vi "SMR_LabVIEW_V4.vi"() -> ()   [LabVIEW 2025]
uses:
  <vilib>/DAQmx/write.llb/DAQmx Write (Analog DBL 1Chan 1Samp).vi
  <vilib>/DAQmx/read.llb/DAQmx Read (Analog 1D DBL NChan 1Samp).vi
  <vilib>/DAQmx/create/channels.llb/DAQmx Create Channel (AI-Temperature-Thermocouple).vi
  <vilib>/DAQmx/create/channels.llb/DAQmx Create Channel (AI-Voltage-Basic).vi
  <vilib>/DAQmx/create/channels.llb/DAQmx Create Channel (AO-Voltage-Basic).vi
  <vilib>/DAQmx/miscellaneous.llb/DAQmx Fill In Error Info.vi
panel:
  in  "Shutdown Valve Command (%)":dbl min=0.0 max=100.0
  out "Valve Command Before Enable (%)":dbl
  out "Valve Output Voltage (V)":dbl
  out "Valve Command Final (%)":dbl
  in  "Valve Output Enable":bool
  in  "Manual Valve Command (%)":dbl min=0.0 max=100.0
  out "Heat Exchanger Pressure History":dbl(graph)
  out "Main Loop Pressure History":T1(graph)
  out "Heat Exchanger Temperature History":cluster{"Waveform":dbl, "Waveform":dbl}(graph)
  out "Main Loop Temeperature History":T2(graph)
  out "Overall Avg Pressure (psi)":dbl
  out "Heat Exchanger Pressure P6 (psi)":dbl
  out "Main Loop Avg Pressure (psi)":dbl
  out "Heat Exchanger Avg Temp (deg C)":dbl
  out "Main Loop Avg Temp (deg C)":dbl
  out "Raw NI9201 \nVoltage Display":T3
  out "Temperature Display":T4
  out "Pressure Display":T5
  in  "Flow Offset Correction (GPM)":dbl=-0.3
  out "Flow History":dbl(graph)
  out "Overall Pressure History":T6(graph)
  out "Overall Temperature History":T7(graph)
  out "Max Loop Pressure (psi)":dbl
  out "Overall Avg Temp (deg C)":dbl
  out "Max Loop Temp (deg C)":dbl
  out "Heat Exchanger Flow (GPM)":dbl
  in  "Loop Period (ms)":dbl=1000.0
  in  "Stop":bool
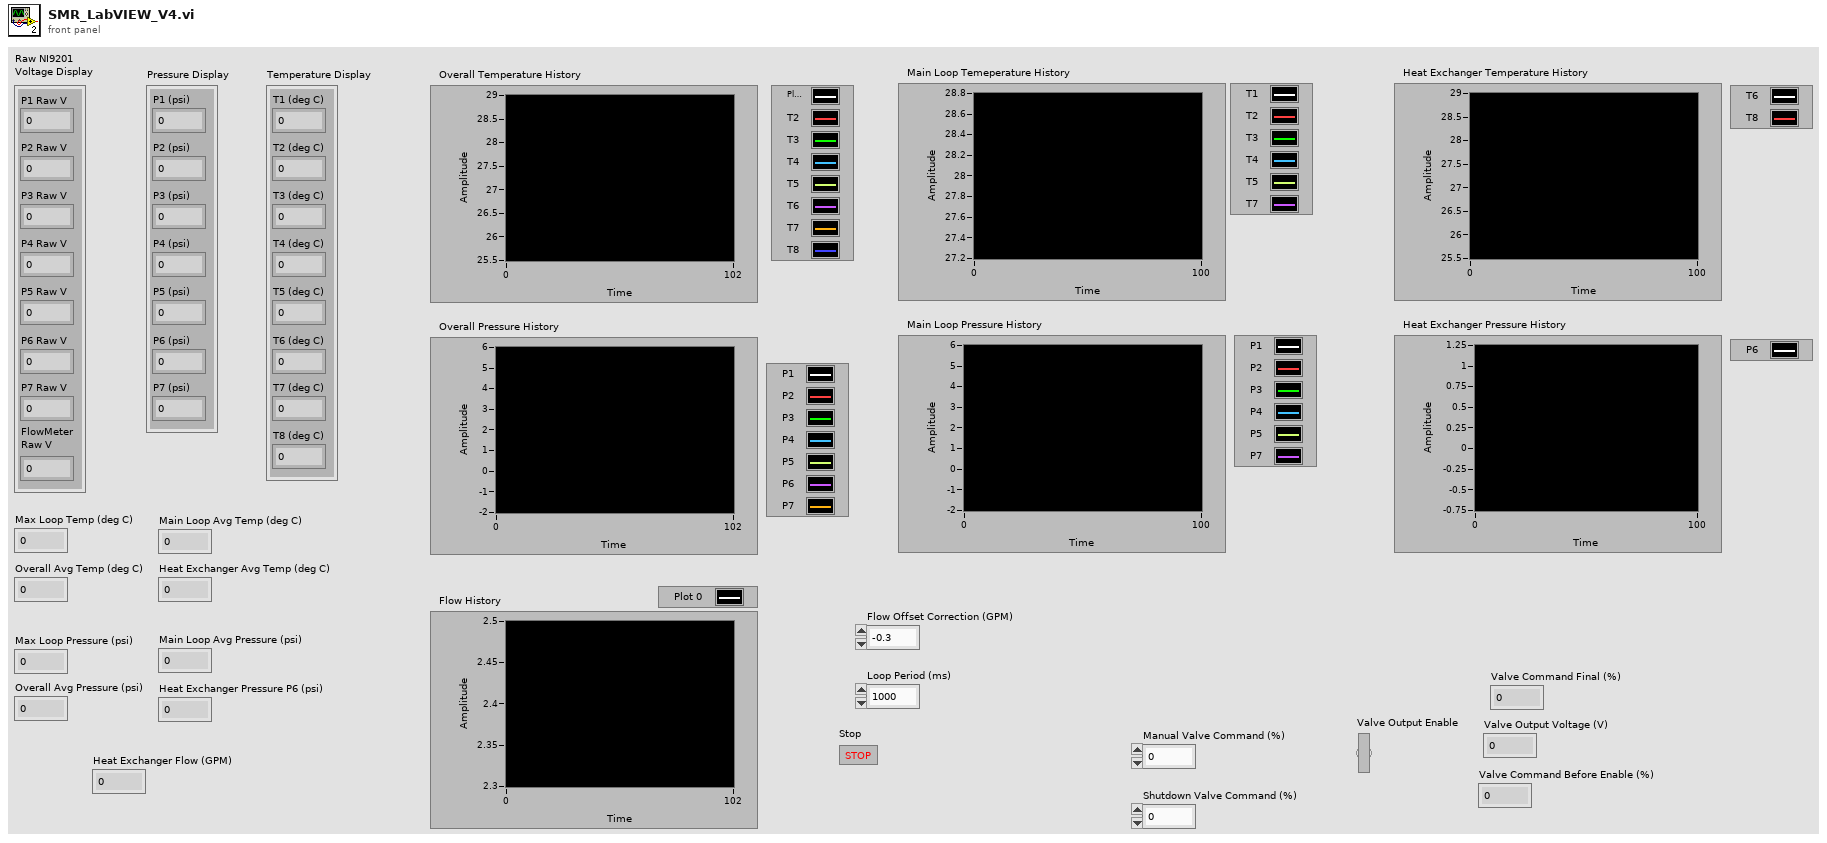
[diagram p1: front panel]
types:
  T1 = cluster{"P1":dbl, "P2":dbl, "P3":dbl, "P4":dbl, "P5":dbl, "P7":dbl}
  T2 = cluster{"Waveform":dbl, "Waveform":dbl, "Waveform":dbl, "Waveform":dbl, "Waveform":dbl, "Waveform":dbl}
  T3 = cluster{"P1 Raw V":dbl, "P2 Raw V":dbl, "P3 Raw V":dbl, "P4 Raw V":dbl, "P5 Raw V":dbl, "P6 Raw V":dbl, "P7 Raw V":dbl, "FlowMeter\nRaw V":dbl}
  T4 = cluster{"T1 (deg C)":dbl, "T2 (deg C)":dbl, "T3 (deg C)":dbl, "T4 (deg C)":dbl, "T5 (deg C)":dbl, "T6 (deg C)":dbl, "T7 (deg C)":dbl, "T8 (deg C)":dbl}
  T5 = cluster{"P1 (psi)":dbl, "P2 (psi)":dbl, "P3 (psi)":dbl, "P4 (psi)":dbl, "P5 (psi)":dbl, "P6 (psi)":dbl, "P7 (psi)":dbl}
  T6 = cluster{"P1":dbl, "P2":dbl, "P3":dbl, "P4":dbl, "P5":dbl, "P6":dbl, "P7":dbl}
  T7 = cluster{"Waveform":dbl, "Waveform":dbl, "Waveform":dbl, "Waveform":dbl, "Waveform":dbl, "Waveform":dbl, "Waveform":dbl, "Waveform":dbl}
  T8 = cluster{"P1":dbl, "P2":dbl, "P3":dbl, "P4":dbl, "P5":dbl, "P6":dbl, "P7":dbl, "Flow":dbl}
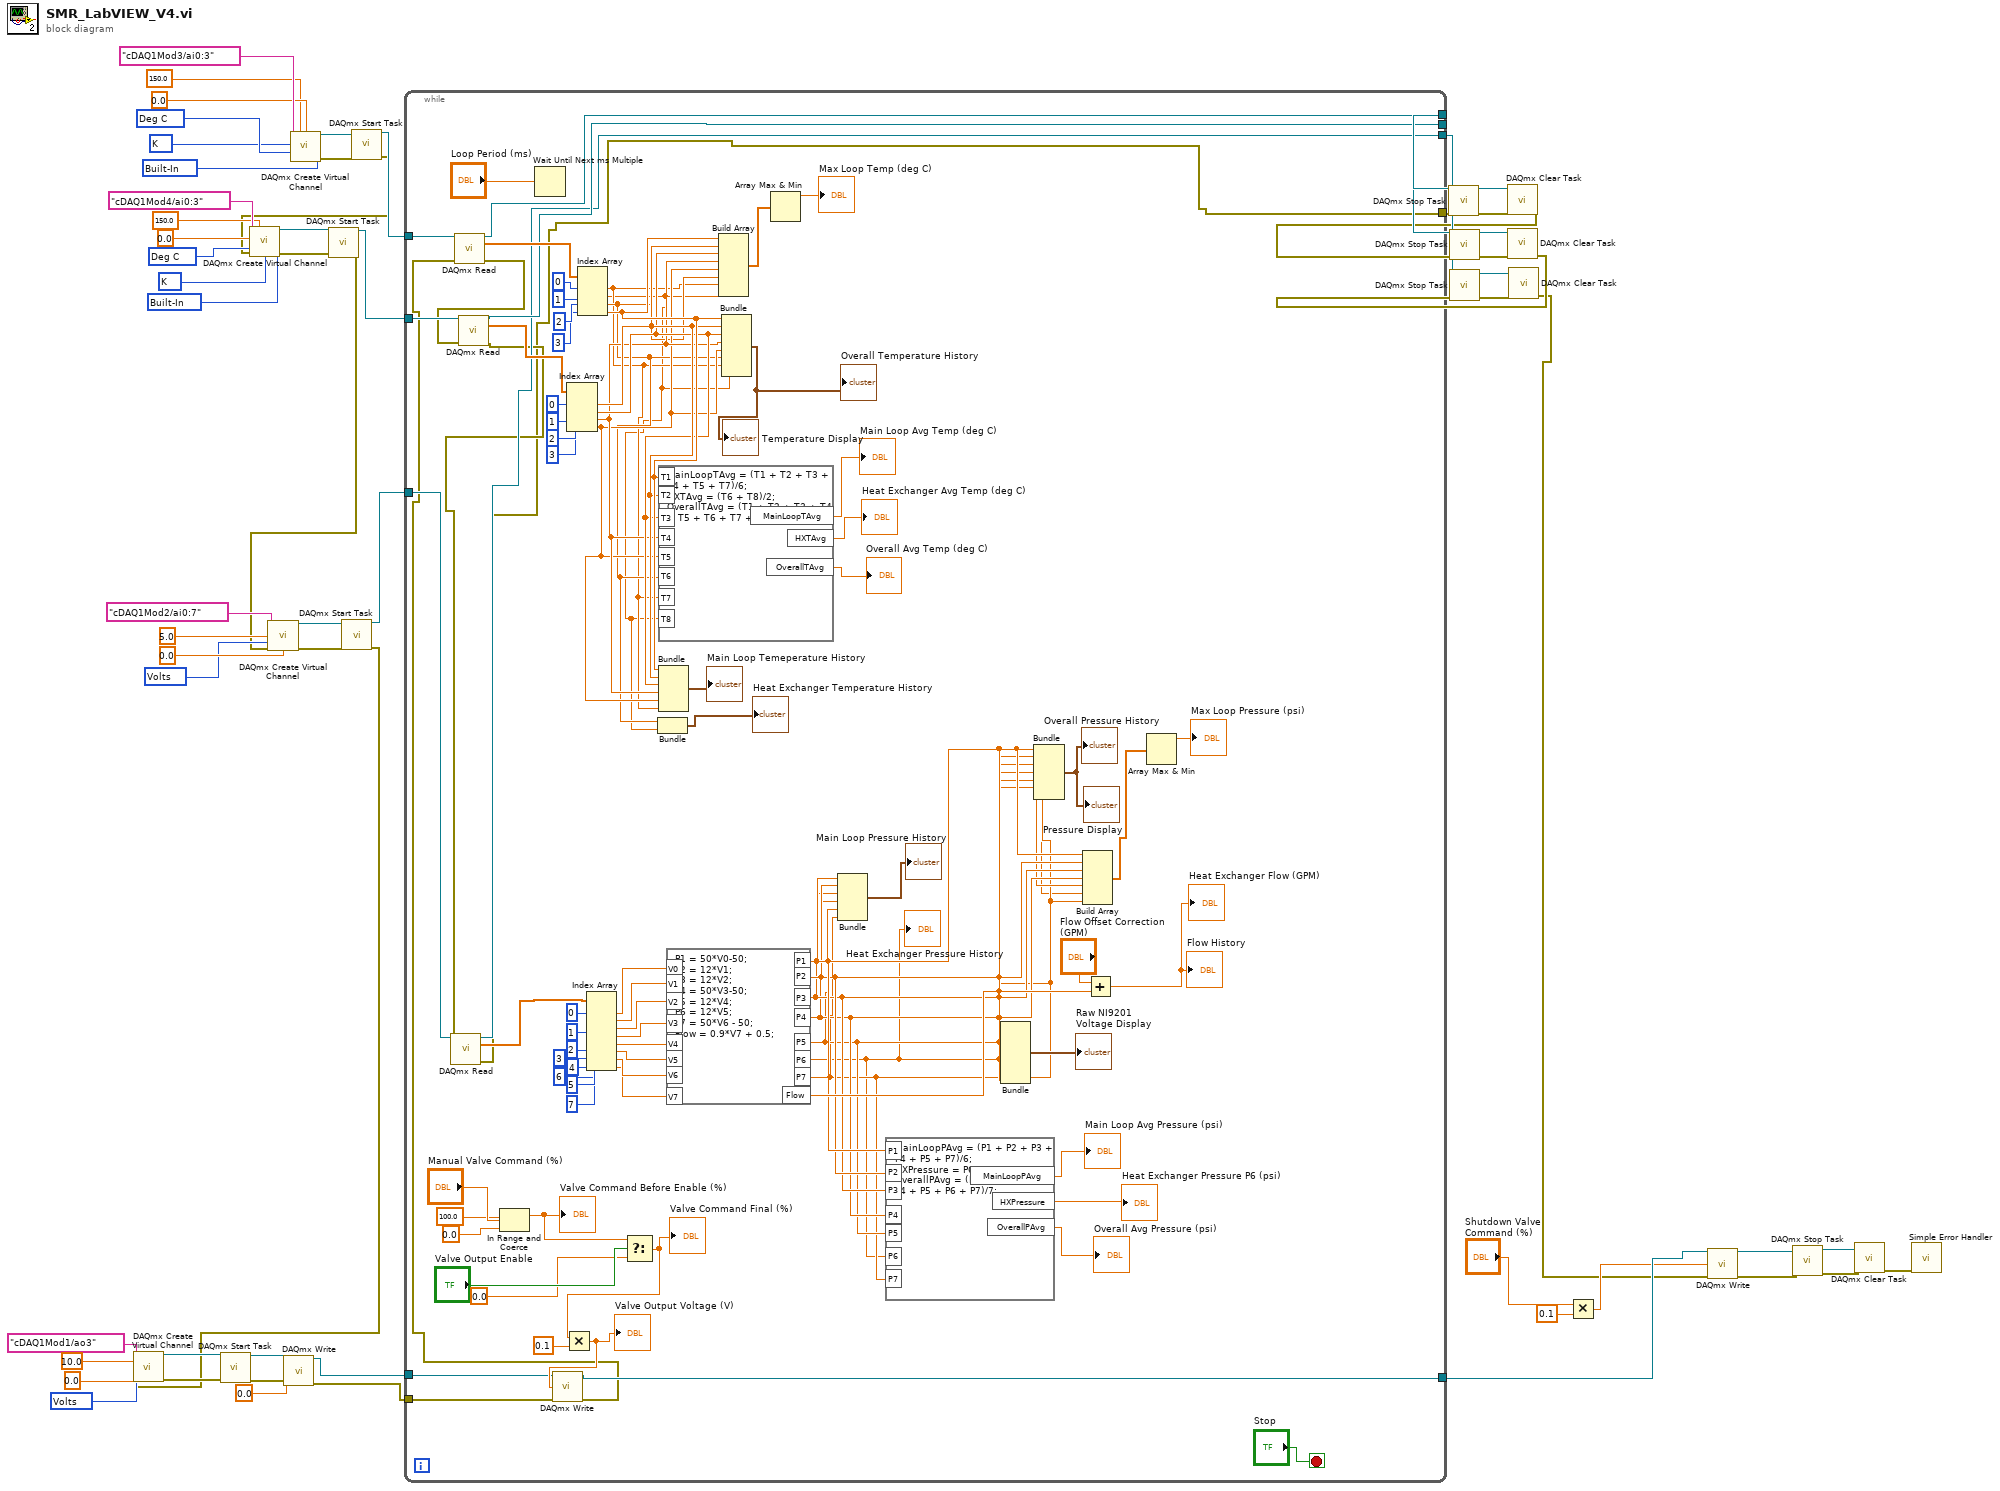
[diagram p0: block diagram]
diagram:
  w19 = 10348 items=["Volts"=10348, "From Custom Scale"=10065] ("units")
  w43 = 10348 items=["Volts"=10348, "From Custom Scale"=10065] ("units")
  w47 = 10200 items=["Built-In"=10200, "Constant Value"=10116, "Channel"=10113] ("cjc source")
  w48 = 10073 items=["J"=10072, "K"=10073, "N"=10077, "R"=10082, "S"=10085, "T"=10086, "B"=10047, "E"=10055] ("thermocouple type")
  w31 = 10143 items=["Deg C"=10143, "Deg F"=10144, "Kelvins"=10325, "Deg R"=10145, "From Custom Scale"=10065] ("units")
  w51 = 10200 items=["Built-In"=10200, "Constant Value"=10116, "Channel"=10113] ("cjc source")
  w52 = 10073 items=["J"=10072, "K"=10073, "N"=10077, "R"=10082, "S"=10085, "T"=10086, "B"=10047, "E"=10055] ("thermocouple type")
  w55 = 10143 items=["Deg C"=10143, "Deg F"=10144, "Kelvins"=10325, "Deg R"=10145, "From Custom Scale"=10065] ("units")
  n1 = call-poly <vilib>:"DAQmx Create Virtual Channel.vi"("maximum value"=150.0, "minimum value"=0.0, "physical channels"=tag "cDAQ1Mod3/ai0:3", "cjc source"=w51, "units"=w55, "thermocouple type"=w52) -> ("task out"=w60:refnum<k21>, "error out"=w59:errorcluster)  [unwired: 8 in]
  n2 = call <vilib>:"DAQmx Start Task.vi"("task/channels in"=w60, "error in"=w59) -> ("task out"=w40:refnum<k21>, "error out"=w30:errorcluster)  [unwired: 12 in]
  n3 = call-poly <vilib>:"DAQmx Create Virtual Channel.vi"("maximum value"=150.0, "minimum value"=0.0, "physical channels"=tag "cDAQ1Mod4/ai0:3", "cjc source"=w47, "units"=w31, "error in"=w30, "thermocouple type"=w48) -> ("task out"=w57:refnum<k21>, "error out"=w56:errorcluster)  [unwired: 7 in]
  n4 = call <vilib>:"DAQmx Start Task.vi"("task/channels in"=w57, "error in"=w56) -> ("task out"=w39:refnum<k21>, "error out"=w29:errorcluster)  [unwired: 12 in]
  n5 = call-poly <vilib>:"DAQmx Create Virtual Channel.vi"("maximum value"=5.0, "minimum value"=0.0, "physical channels"=tag "cDAQ1Mod2/ai0:7", "units"=w43, "error in"=w29) -> ("task out"=w42:refnum<k21>, "error out"=w41:errorcluster)  [unwired: 9 in]
  n6 = call <vilib>:"DAQmx Start Task.vi"("task/channels in"=w42, "error in"=w41) -> ("task out"=w38:refnum<k21>, "error out"=w6:errorcluster)  [unwired: 12 in]
  n7 = call-poly <vilib>:"DAQmx Create Virtual Channel.vi"("maximum value"=10.0, "minimum value"=0.0, "physical channels"=tag "cDAQ1Mod1/ao3", "units"=w19, "error in"=w6) -> ("task out"=w18:refnum<k21>, "error out"=w17:errorcluster)  [unwired: 9 in]
  n8 = call <vilib>:"DAQmx Start Task.vi"("task/channels in"=w18, "error in"=w17) -> ("task out"=w16:refnum<k21>, "error out"=w14:errorcluster)  [unwired: 12 in]
  n9 = call-poly <vilib>:"DAQmx Write.vi"("task/channels in"=w16, "data"=0.0, "error in"=w14) -> ("task out"=w13:refnum<k21>, "error out"=w5:errorcluster)  [unwired: 10 in, 1 out]
  n10 = while {
    tunnel: w40 -> [w144]
    tunnel: w39 -> [w143]
    tunnel: w38 -> [w130]
    tunnel: [w111] -> w37
    tunnel: [w110] -> w36
    tunnel: [w109] -> w35
    tunnel: [w106] -> w28
    tunnel: w13 -> [w65]
    tunnel: [w64] -> w10
    tunnel: w5 -> [w63]
    stop <- "Stop" stop-if-true
    n11 = In Range and Coerce(upper limit=100.0, x="Manual Valve Command (%)", lower limit=0.0) -> (coerced(x)=w69:dbl)  [unwired: 1 out]
    "Valve Command Before Enable (%)" <- w69
    n12 = Wait Until Next ms Multiple(millisecond multiple="Loop Period (ms)") -> ()  [unwired: 1 out]
    n13 = Select(t=w69, s="Valve Output Enable", f=0.0) -> (s? t:f=w67:dbl)
    "Valve Command Final (%)" <- w67
    n14 = Multiply(x=w67, y=0.1) -> (x*y=w66:dbl)
    "Valve Output Voltage (V)" <- w66
    n15 = call-poly <vilib>:"DAQmx Write.vi"("task/channels in"=w65, "data"=w66, "error in"=w63) -> ("task out"=w64:refnum<k21>, "error out"=w62:errorcluster)  [unwired: 10 in, 1 out]
    n16 = call-poly <vilib>:"DAQmx Read.vi"("task/channels in"=w144, "error in"=w62) -> ("task out"=w111:refnum<k21>, "data"=w134:dbl[], "error out"=w108:errorcluster)  [unwired: 11 in]
    n17 = call-poly <vilib>:"DAQmx Read.vi"("task/channels in"=w143, "error in"=w108) -> ("task out"=w110:refnum<k21>, "data"=w133:dbl[], "error out"=w107:errorcluster)  [unwired: 11 in]
    n18 = call-poly <vilib>:"DAQmx Read.vi"("task/channels in"=w130, "error in"=w107) -> ("task out"=w109:refnum<k21>, "data"=w121:dbl[], "error out"=w106:errorcluster)  [unwired: 11 in]
    n19 = Index Array(array=w133, index #1=0 ("index"), index #2=1 ("index"), index #3=2 ("index"), index #4=3 ("index")) -> (element #1=w91:dbl, element #2=w90:dbl, element #3=w89:dbl, element #4=w88:dbl)
    n20 = Index Array(array=w134, index #1=0 ("index"), index #2=1 ("index"), index #3=2 ("index"), index #4=3 ("index")) -> (element #1=w85:dbl, element #2=w84:dbl, element #3=w86:dbl, element #4=w92:dbl)
    n21 = Index Array(array=w121, index #1=0 ("index"), index #2=1 ("index"), index #3=2 ("index"), index #4=3 ("index"), index #5=4 ("index"), index #6=5 ("index"), index #7=6 ("index"), index #8=7 ("index")) -> (element #1=w120:dbl, element #2=w119:dbl, element #3=w118:dbl, element #4=w117:dbl, element #5=w116:dbl, element #6=w115:dbl, element #7=w114:dbl, element #8=w113:dbl)
    n22 = Bundle("Waveform"=w86, "Waveform"=w84) -> (→"Heat Exchanger Temperature History":cluster{"Waveform":dbl, "Waveform":dbl})  [unwired: 1 in]
    n23 = formula code="MainLoopTAvg = (T1 + T2 + T3 + T4 + T5 + T7)/6;\nHXTAvg = (T6 + T8)/2;\nOverallTAvg = (T1 + T2 + T3 + T4 + T5 + T6 + T7 + T8)/8;"("T1"=w92, "T2"=w91, "T3"=w90, "T4"=w89, "T5"=w88, "T6"=w86, "T7"=w85, "T8"=w84) -> ("MainLoopTAvg"=→"Main Loop Avg Temp (deg C)":dbl, "HXTAvg"=→"Heat Exchanger Avg Temp (deg C)":dbl, "OverallTAvg"=→"Overall Avg Temp (deg C)":dbl)
    n24 = Bundle("Waveform"=w92, "Waveform"=w91, "Waveform"=w90, "Waveform"=w89, "Waveform"=w88, "Waveform"=w85) -> (→"Main Loop Temeperature History":T2)  [unwired: 1 in]
    n25 = formula code="P1 = 50*V0-50;\nP2 = 12*V1;\nP3 = 12*V2;\nP4 = 50*V3-50;\nP5 = 12*V4;\nP6 = 12*V5; \nP7 = 50*V6 - 50;\nFlow = 0.9*V7 + 0.5;"("V0"=w120, "V1"=w119, "V2"=w118, "V3"=w117, "V4"=w116, "V5"=w115, "V6"=w114, "V7"=w113) -> ("P1"=w82:dbl, "P2"=w81:dbl, "P3"=w80:dbl, "P4"=w79:dbl, "P5"=w78:dbl, "P6"=w75:dbl, "P7"=w77:dbl, "Flow"=w100:dbl)
    "Heat Exchanger Pressure History" <- w75
    n26 = Build Array(w92, w91, w90, w89, w88, w86, w85, w84) -> (w131:dbl[])
    n27 = Bundle("Waveform"=w92, "Waveform"=w91, "Waveform"=w90, "Waveform"=w89, "Waveform"=w88, "Waveform"=w86, "Waveform"=w85, "Waveform"=w84) -> (→"Overall Temperature History" →"Temperature Display":T7)  [unwired: 1 in]
    n28 = Array Max & Min(array=w131) -> (max value=→"Max Loop Temp (deg C)":dbl)  [unwired: 3 out]
    n29 = Bundle("P1"=w82, "P2"=w81, "P3"=w80, "P4"=w79, "P5"=w78, "P7"=w77) -> (→"Main Loop Pressure History":T1)  [unwired: 1 in]
    n30 = formula code="MainLoopPAvg = (P1 + P2 + P3 + P4 + P5 + P7)/6;\nHXPressure = P6;\nOverallPAvg = (P1 + P2 + P3 + P4 + P5 + P6 + P7)/7;"("P1"=w82, "P2"=w81, "P3"=w80, "P4"=w79, "P5"=w78, "P6"=w75, "P7"=w77) -> ("MainLoopPAvg"=→"Main Loop Avg Pressure (psi)":dbl, "HXPressure"=→"Heat Exchanger Pressure P6 (psi)":dbl, "OverallPAvg"=→"Overall Avg Pressure (psi)":dbl)
    n31 = Bundle("P1"=w82, "P2"=w81, "P3"=w80, "P4"=w79, "P5"=w78, "P6"=w75, "P7"=w77, "Flow"=w100) -> (→"Raw NI9201 \nVoltage Display":T8)  [unwired: 1 in]
    n32 = Bundle("P1"=w82, "P2"=w81, "P3"=w80, "P4"=w79, "P5"=w78, "P6"=w75, "P7"=w77) -> (→"Overall Pressure History" →"Pressure Display":T6)  [unwired: 1 in]
    n33 = Build Array(w82, w81, w80, w79, w78, w75, w77) -> (w103:dbl[])
    n34 = Add(x="Flow Offset Correction (GPM)", y=w100) -> (x+y=→"Heat Exchanger Flow (GPM)" →"Flow History":dbl)
    n35 = Array Max & Min(array=w103) -> (max value=→"Max Loop Pressure (psi)":dbl)  [unwired: 3 out]
  }
  n36 = call <vilib>:"DAQmx Stop Task.vi"("task/channels in"=w37, "error in"=w28) -> ("task out"=w34:refnum<k21>, "error out"=w27:errorcluster)  [unwired: 12 in]
  n37 = call <vilib>:"DAQmx Clear Task.vi"("task in"=w34, "error in"=w27) -> ("error out"=w26:errorcluster)  [unwired: 13 in]
  n38 = call <vilib>:"DAQmx Stop Task.vi"("task/channels in"=w36, "error in"=w26) -> ("task out"=w33:refnum<k21>, "error out"=w25:errorcluster)  [unwired: 12 in]
  n39 = call <vilib>:"DAQmx Clear Task.vi"("task in"=w33, "error in"=w25) -> ("error out"=w24:errorcluster)  [unwired: 13 in]
  n40 = call <vilib>:"DAQmx Stop Task.vi"("task/channels in"=w35, "error in"=w24) -> ("task out"=w32:refnum<k21>, "error out"=w23:errorcluster)  [unwired: 12 in]
  n41 = call <vilib>:"DAQmx Clear Task.vi"("task in"=w32, "error in"=w23) -> ("error out"=w4:errorcluster)  [unwired: 13 in]
  n42 = Multiply(x="Shutdown Valve Command (%)", y=0.1) -> (x*y=w9:dbl)
  n43 = call-poly <vilib>:"DAQmx Write.vi"("task/channels in"=w10, "data"=w9, "error in"=w4) -> ("task out"=w8:refnum<k21>, "error out"=w3:errorcluster)  [unwired: 10 in, 1 out]
  n44 = call <vilib>:"DAQmx Stop Task.vi"("task/channels in"=w8, "error in"=w3) -> ("task out"=w7:refnum<k21>, "error out"=w2:errorcluster)  [unwired: 12 in]
  n45 = call <vilib>:"DAQmx Clear Task.vi"("task in"=w7, "error in"=w2) -> ("error out"=w1:errorcluster)  [unwired: 13 in]
  n46 = call <vilib>:"Simple Error Handler.vi"("error in (no error)"=w1) -> ()  [unwired: 4 in, 5 out]
